vi "Get Flow Rate.vi"(8 "error in (no error)":errorcluster, 11 "Aalborg GFC17 in":refnum<class "Aalborg GFC17.lvclass">) -> (0 "error out":errorcluster, 1 "Flow Rate Units":T1, 2 "Flow Rate":dbl, 3 "Aalborg GFC17 out":refnum<class "Aalborg GFC17.lvclass">)   [LabVIEW 2011, in "Aalborg GFC17.lvclass"]
uses:
  Aalborg GFC17.lvclass
  Mass Flow Controller/Flow Rate Units.ctl
  Aalborg GFC17.lvclass/Aalborg GFC17.ctl
  <vilib>/DAQmx/read.llb/DAQmx Read (Analog DBL 1Chan 1Samp).vi
  <vilib>/DAQmx/miscellaneous.llb/DAQmx Fill In Error Info.vi
  Mass Flow Controller/Mass Flow Controller.lvclass
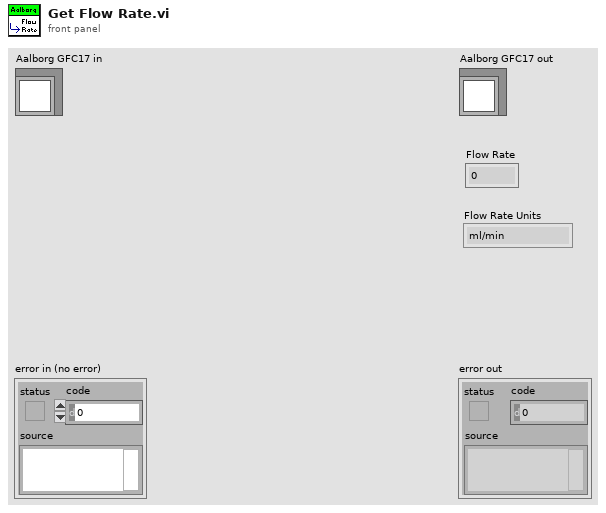
[diagram p1: front panel]
types:
  T1 = typedef "Mass Flow Controller.lvclass/Flow Rate Units.ctl" = enum16{"ml/min"}
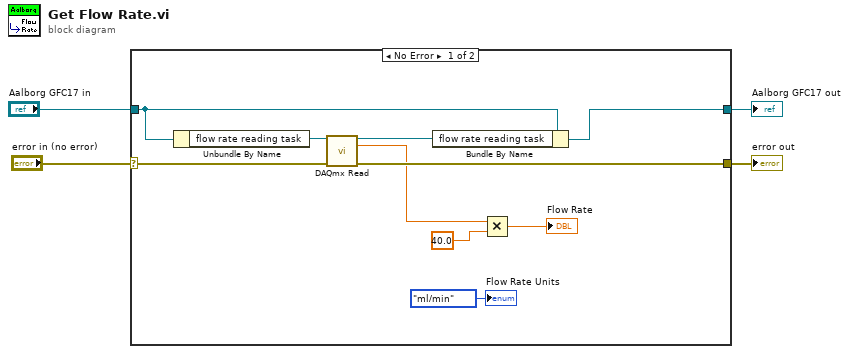
[diagram p0: block diagram]
diagram:
  n1 = case shown="No Error" "error in (no error)" {
    selector: "error in (no error)" -> [w13 w16]
    tunnel: [w7 w16] -> w3
    tunnel: [w9 w15] -> w1
    tunnel: "Aalborg GFC17 in" -> [w11 w15]
    frame No Error {
      n2 = Unbundle By Name(w11) -> ("flow rate reading task"=w12:refnum<k21>)
      n3 = call-poly <vilib>:"DAQmx Read.vi"("task/channels in"=w12, "error in"=w13) -> ("task out"=w10:refnum<k21>, "data"=w6:dbl, "error out"=w7:errorcluster)  [unwired: 11 in]
      n4 = Bundle By Name(cluster=w11, "flow rate reading task"=w10) -> (w9:refnum<class "Aalborg GFC17.lvclass">)
      n5 = Multiply(x=w6, y=40.0) -> (x*y=→"Flow Rate":dbl)
      "Flow Rate Units" <- Flow_Rate_Units."ml/min" ("Flow Rate Units")
    }
    frame Error {
    }
  }
  "error out" <- w3
  "Aalborg GFC17 out" <- w1
